vi "real time imaging v2.vi"() -> ()   [LabVIEW 2016]
uses:
  C:/Laser generated ultrasound/Labview/Kinesis Control/Thorlabs.MotionControl.KCube.BrushlessMotorCLI.dll
  Thorlabs.MotionControl.KCube.BrushlessMotorCLI.dll
  <vilib>/Analysis/3filter.llb/Filter Passband Type.ctl
  <vilib>/Analysis/baseanly.llb/Mean (DBL).vi
  <vilib>/Analysis/baseanly.llb/Real A x B.vi
  <vilib>/Utility/file.llb/Write To Spreadsheet File (DBL).vi
  <instrlib>/niScope/Acquire/Fetch/niScope Fetch.vi
  <vilib>/Analysis/Matrix/Numeric/Conversions/Array To Matrix - RA2.vi
  <vilib>/Analysis/Matrix/Numeric/Conversions/Matrix To Array - RM.vi
  <vilib>/Analysis/3filter.llb/Butterworth Filter (DBL).vi
  <instrlib>/niScope/Acquire/Fetch/niScope Multi Fetch.vi
  C:/Laser generated ultrasound/Labview/Kinesis Control/Thorlabs.MotionControl.Controls.dll
  Thorlabs.MotionControl.Controls.dll
  <vilib>/Analysis/NI_AALBase.lvlib
  <vilib>/Analysis/Matrix/NI_Matrix.lvlib
  <vilib>/Analysis/NI_AALPro.lvlib
panel:
  in  "stop":bool
  in  "Tab Control":T1(tab)
  in  "File Location":string="C:\\Laser generated ultrasound\\Labview\\Kinesis Control\\test data"
  in  "File name":string="scan_1"
  in  "SerialNumber":string="28251512"
  in  "Scan Length (mm)":dbl=20.0
  in  "Pullback speed (mm/s)":dbl=40.0
  in  "Repetition rate (Hz)":dbl=100.0
  in  "vertical range (V)":dbl=0.5 min=0.0 max=10.0 step=0.5
  in  "Depth (mm)":i32=15
  in  "Start acquisition":bool
  out "Number of samples":dbl
  out "number of a-lines":dbl
  in  "Apply frequency filter":bool
  in  "High Cutoff (MHz)":dbl=45.0
  in  "Low Cutoff (MHz)":dbl=1.0
  in  "Number of points":i32=150
  in  "Exponent":dbl=2.5
  out "spare a-lines":dbl
  out "?":cluster{dbl[], dbl[]}(graph)
  in  "Preview A-line?":bool
  in  "Start save":bool
  out "Intensity Graph":dbl[][](graph)
  in  "Stop save":bool
  out "Acquiring Data":bool
  in  "KCubeBrushlessControl":refnum<k24>(container)
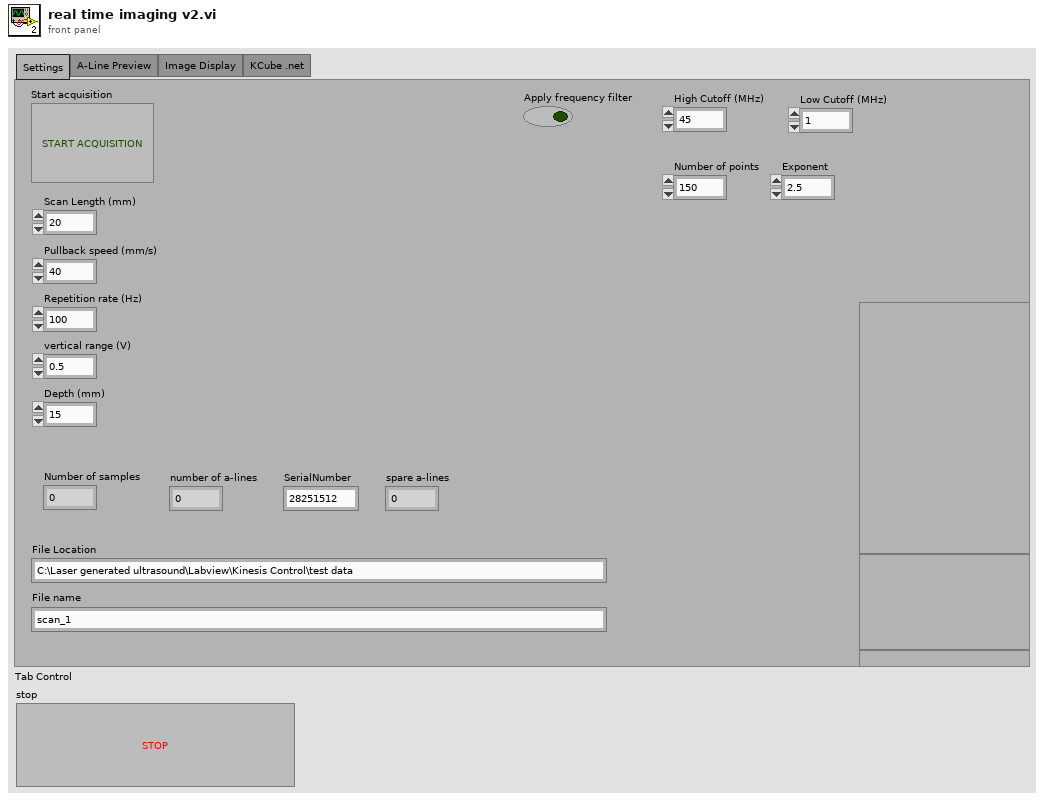
[diagram p1: front panel]
types:
  T1 = enum32{"Settings", "A-Line Preview", "Image Display", "KCube .net"}
  T2 = typedef "NI_AALBase.lvlib/Filter Passband Type.ctl" = enum32{"Lowpass", "Highpass", "Bandpass", "Bandstop"}
  T3 = typedef "NI_Matrix.lvlib/RealMatrix.ctl" = dbl[][]
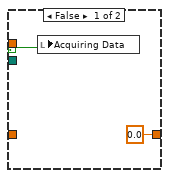
[diagram p8: hidden frame]
diagram:
  n1 = flat-sequence {
    tunnel: [w115] -> w72
    tunnel: [w114] -> w70
    tunnel: [w113] -> w68
    tunnel: [w111] -> w66
    tunnel: [w110] -> w64
    tunnel: [w98] -> w62
    tunnel: [w99] -> w60
    tunnel: ["Scan Length (mm)"] -> w58
    tunnel: ["Pullback speed (mm/s)"] -> w56
    tunnel: [w82] -> w54
    tunnel: ["File Location"] -> w53
    tunnel: ["File name"] -> w52
    tunnel: [w91] -> w44
    tunnel: [w91] -> w41
    tunnel: [w84] -> w11
    tunnel: ["Depth (mm)"] -> w6
    tunnel: [w82] -> w5
    tunnel: [w78] -> w4
    tunnel: [w77] -> w3
    tunnel: [w75] -> w2
    tunnel: [w73] -> w1
    tunnel: w72 -> [w181]
    tunnel: [w181] -> w71
    tunnel: w70 -> [w180]
    tunnel: [w180] -> w69
    tunnel: w68 -> [w179]
    tunnel: [w179] -> w67
    tunnel: w66 -> [w178]
    tunnel: [w178] -> w65
    tunnel: w64 -> [w177]
    tunnel: [w177] -> w63
    tunnel: w62 -> [w176]
    tunnel: [w176] -> w61
    tunnel: w60 -> [w175]
    tunnel: [w175] -> w59
    tunnel: w58 -> [w174]
    tunnel: [w174] -> w57
    tunnel: w56 -> [w173]
    tunnel: [w173] -> w55
    tunnel: w54 -> [w171]
    tunnel: w53 -> [w143]
    tunnel: w52 -> [w142]
    tunnel: w44 -> [w150]
    tunnel: [w150] -> w43
    tunnel: w41 -> [w148]
    tunnel: w11 -> [_]
    tunnel: [w136] -> w10
    tunnel: w6 -> [w140]
    tunnel: w5 -> [w139]
    tunnel: w4 -> [w135]
    tunnel: w3 -> [w134]
    tunnel: w2 -> [w133]
    tunnel: w1 -> [w130]
    tunnel: w71 -> [w194]
    tunnel: w69 -> [w189]
    tunnel: w67 -> [w190]
    tunnel: [w194] -> w51
    tunnel: [w189] -> w50
    tunnel: [w190] -> w49
    tunnel: w65 -> [w188]
    tunnel: w63 -> [w187]
    tunnel: [w188] -> w48
    tunnel: [w187] -> w47
    tunnel: [w186] -> w46
    tunnel: w61 -> [w185]
    tunnel: [w185] -> w45
    tunnel: w59 -> [w186]
    tunnel: w57 -> [_]
    tunnel: w55 -> [w184]
    tunnel: w43 -> [w183]
    tunnel: [w183] -> w42
    tunnel: w10 -> [w182]
    tunnel: [w182] -> w9
    tunnel: w51 -> [w207]
    tunnel: [w207] -> w40
    tunnel: w50 -> [w206]
    tunnel: [w206] -> w38
    tunnel: w49 -> [w205]
    tunnel: [w205] -> w36
    tunnel: w48 -> [w204]
    tunnel: [w203] -> w34
    tunnel: w47 -> [w202]
    tunnel: [w201] -> w32
    tunnel: w46 -> [w200]
    tunnel: [w197] -> w30
    tunnel: w45 -> [w199]
    tunnel: [w196] -> w28
    tunnel: w42 -> [w198]
    tunnel: w9 -> [w195]
    tunnel: [w195] -> w8
    tunnel: w40 -> [w237]
    tunnel: [w237] -> w39
    tunnel: w38 -> [w236]
    tunnel: [w236] -> w37
    tunnel: w36 -> [w235]
    tunnel: [w235] -> w35
    tunnel: w34 -> [w234]
    tunnel: [w234] -> w33
    tunnel: w32 -> [w233]
    tunnel: [w233] -> w31
    tunnel: w30 -> [w232]
    tunnel: [w230] -> w29
    tunnel: w28 -> [w231]
    tunnel: [w229] -> w27
    tunnel: [w225] -> w26
    tunnel: w8 -> [w224]
    tunnel: [w224] -> w7
    tunnel: w39 -> [w249]
    tunnel: w37 -> [w247]
    tunnel: w35 -> [w248]
    tunnel: [w249] -> w25
    tunnel: [w247] -> w23
    tunnel: [w248] -> w21
    tunnel: w33 -> [w246]
    tunnel: w31 -> [w245]
    tunnel: [w246] -> w19
    tunnel: [w245] -> w17
    tunnel: [w241] -> w15
    tunnel: [w240] -> w13
    tunnel: w29 -> [w244]
    tunnel: w27 -> [w243]
    tunnel: w26 -> [w242]
    tunnel: w7 -> [w239]
    tunnel: w25 -> [w543]
    tunnel: [w543] -> w24
    tunnel: w23 -> [w542]
    tunnel: [w542] -> w22
    tunnel: w21 -> [w541]
    tunnel: [w541] -> w20
    tunnel: w19 -> [w540]
    tunnel: [w540] -> w18
    tunnel: w17 -> [w539]
    tunnel: [w539] -> w16
    tunnel: w15 -> [w538]
    tunnel: [w538] -> w14
    tunnel: w13 -> [w537]
    tunnel: [w537] -> w12
    tunnel: w24 -> [w545]
    tunnel: w22 -> [w544]
    tunnel: w20 -> [_]
    tunnel: w18 -> [w549]
    tunnel: w16 -> [w548]
    tunnel: w14 -> [w547]
    tunnel: w12 -> [w546]
    frame #0 {
      # "spare a lines are acquired before the motor moves\nthink of this as a buffer to remove them\n0.05 estimated empirically"
      # "add extra a-lines as a buffer"
      # "calculate number of a-lines"
      # "Initiialise data array"
      # "round trip"
      # "speed of sound"
      # "convert depth to samples"
      # "convert to metre"
      # "Intialise all the equipment\n1. Motor\n2. Trigger\n3. Acquisition"
      n2 = Multiply(x=1500 ("y"), y=1e-08) -> (x*y=w103:dbl)
      n3 = local read "Pullback speed (mm/s)"() -> (w88:dbl)
      n4 = local read "Scan Length (mm)"() -> (w89:dbl)
      n5 = call "pulse_init.vi"("Repetition rate"="Repetition rate (Hz)") -> ("error out"=w110:errorcluster, "Refnum out"=w111:refnum<k21>)  [unwired: 9 in]
      n6 = local read "Repetition rate (Hz)"() -> (w87:dbl)
      n7 = Divide(x="Depth (mm)", y=1000) -> (x/y=w102:dbl)
      n8 = Multiply(x=w102, y=2.0) -> (x*y=w100:dbl)
      n9 = property class="KCubeBrushlessControl"(reference="KCubeBrushlessControl", "SerialNumber"="SerialNumber") -> (reference out=w119:refnum<k24>, error out=w118:errorcluster)  [unwired: 1 in]
      n10 = Divide(x=w100, y=w103) -> (x/y=w105:dbl)
      n11 = local read "Scan Length (mm)"() -> (w79:dbl)
      n12 = local read "Pullback speed (mm/s)"() -> (w77:dbl)
      n13 = Round Toward +Infinity(x=w105) -> (ceil(x): smallest int >= x=w82:dbl)
      "Number of samples" <- w82
      n14 = Initialize Array(0.0 ("element"), w82) -> (w92:dbl[])
      n15 = for {
        N: w82 -> [_]
        shift-right: [w127] -> w91
        shift-left: w92 -> [w126]
        i -> [w125]
        # "Create time axis"
        n16 = To Double Precision Float(number=w125) -> (double precision float=w124:dbl)
        n17 = Multiply(x=w124, y=1e-08) -> (x*y=w122:dbl)
        n18 = Replace Array Subset(array=w126, new element=w122, index=w125) -> (w127:dbl[])
      }
      n19 = Divide(x=w89, y=w88) -> (x/y=w86:dbl)
      n20 = local read "Repetition rate (Hz)"() -> (w75:dbl)
      n21 = Multiply(x=w86, y=w87) -> (x*y=w85:dbl)
      n22 = call "scope_init.vi"("Num Samples"=w82, "vertical range"="vertical range (V)", "Averages"=1) -> ("error out"=w98:errorcluster, "IVI Refnum out"=w99:refnum<k15>)  [unwired: 7 in]
      n23 = Initialize Array(0.0 ("element"), w82, w85) -> (w84:dbl[][])
      n24 = invoke class="KCubeBrushlessControl" method="CreateDevice"(reference=w119, error in=w118) -> (reference out=w117:refnum<k24>, error out=w116:errorcluster)  [unwired: 1 in, 1 out]
      n25 = Divide(x=w77, y=w75) -> (x/y=w80:dbl)
      n26 = Divide(x=w79, y=w80) -> (x/y=w81:dbl)
      n27 = Multiply(x=w75, y=0.05 ("x")) -> (x*y=w74:dbl)
      n28 = property class="KCubeBrushlessControl"(reference=w117, error in=w116) -> (reference out=w115:refnum<k24>, error out=w114:errorcluster, "Device"=w113:refnum<k24>)
      n29 = Round Toward +Infinity(x=w74) -> (ceil(x): smallest int >= x=w73:dbl)
      "spare a-lines" <- w73
      n30 = Add(x=w81, y=w73) -> (x+y=w78:dbl)
      "number of a-lines" <- w78
    }
    frame #1 {
      w128 = "\r"
      w131 = "\t"
      # "Calculate spare a-lines before move"
      # "Save the header file"
      # "Initialise the data matrix"
      # "Initialise the data matrix\nSave the Header file"
      n31 = local read "Repetition rate (Hz)"() -> (w158:dbl)
      n32 = local read "Number of samples"() -> (w164:dbl)
      n33 = local read "number of a-lines"() -> (w161:dbl)
      n34 = local read "Scan Length (mm)"() -> (w155:dbl)
      n35 = local read "Pullback speed (mm/s)"() -> (w152:dbl)
      n36 = Number To Decimal String(number=w164) -> (decimal integer string=w163:string)  [unwired: 1 in]
      n37 = Number To Decimal String(number=w158) -> (decimal integer string=w157:string)  [unwired: 1 in]
      n38 = Number To Decimal String(number=w161) -> (decimal integer string=w160:string)  [unwired: 1 in]
      n39 = Number To Decimal String(number=w155) -> (decimal integer string=w154:string)  [unwired: 1 in]
      n40 = Concatenate Strings(w143, "\\" ("string"), w142, "_hdr.txt" ("string")) -> (w169:string)
      n41 = Divide(x=w140, y=w139) -> (x/y=w138:dbl)
      n42 = Number To Decimal String(number=w152) -> (decimal integer string=w151:string)  [unwired: 1 in]
      n43 = Concatenate Strings(w143, "\\" ("string"), w142, "_taxis.txt" ("string")) -> (w147:string)
      n44 = Divide(x=w134, y=w133) -> (x/y=w141:dbl)
      n45 = String To Path(string=w147) -> (path=w144:path)
      n46 = property on="Intensity Graph" class="IntGraph (strict)"("XScale.Multiplier"=w141, "YScale.Multiplier"=w138) -> ()  [unwired: 2 in, 2 out]
      n47 = Number To Decimal String(number=w130) -> (decimal integer string=w129:string)  [unwired: 1 in]
      n48 = property on="Intensity Graph" class="IntGraph (strict)"("ZScale.MarkerVals[]"=cluster{dbl, u32}[] [{0.0, 0}, {-1.0, 16711680}, {-2.0, 16744192}, {-3.0, 16777087}, {-5.0, 16777215}] ("Z Scale.Marker Values[]")) -> ()  [unwired: 2 in, 2 out]
      n49 = Initialize Array(0.0 ("element"), w171, w135) -> (w136:dbl[][])
      n50 = call-poly <vilib>:"Write To Spreadsheet File.vi"("format (%.3f)"="%#g", "1D data"=w148, "file path (dialog if empty)"=w144) -> ()  [unwired: 5 in, 1 out]
      n51 = Concatenate Strings("Samples per A-line" ("string"), w131, w163, w128, "Number of A-lines" ("string"), w131, w160, w128, "Repetition rate (Hz)" ("string"), w131, w157, w128, "Scan length (mm)" ("string"), w131, w154, w128, "Pullback speed (mm/s)" ("string"), w131, w151, w128, "Spare a-line" ("string"), w131, w129, w128) -> (w166:string)
      n52 = String To Path(string=w169) -> (path=w170:path)
      n53 = Write to Text File(file (use dialog)=w170, text=w166) -> ()  [unwired: 2 in, 3 out]
    }
    frame #2 {
      # "Initial data array"
      # "Home the motor"
      n54 = invoke class="KCubeBrushlessMotor" method="Home"(reference=w190, error in=w189, "waitTimeout"=50000) -> ()  [unwired: 1 in, 4 out]
      n55 = invoke class="KCubeBrushlessMotor" method="SetVelocityParams"(reference=w190, error in=w189, "maxVelocity"=w184, "acceleration"=999.7) -> ()  [unwired: 1 in, 5 out]
      n56 = Wait (ms)(milliseconds to wait=u32 1000) -> ()  [unwired: 1 out]
    }
    frame #3 {
      # "A-line display for positioning"
      n57 = while {
        tunnel: w204 -> [w222]
        tunnel: w202 -> [w221]
        tunnel: [w222] -> w203
        tunnel: [w221] -> w201
        tunnel: w200 -> [w218]
        tunnel: w199 -> [w217]
        tunnel: w198 -> [w212]
        tunnel: [w209] -> w197
        tunnel: [w208] -> w196
        stop <- "Start acquisition" stop-if-true
        n58 = local read "Number of samples"() -> (w220:dbl)
        n59 = call <instrlib>:"niScope Initiate Acquisition.vi"("instrument handle"=w218, "error in"=w217) -> ("instrument handle out"=w216:refnum<k15>, "error out"=w215:errorcluster)  [unwired: 12 in]
        n60 = call-poly <instrlib>:"niScope Fetch (poly).vi"("error in"=w215, "numSamples"=w220, "channels"="0", "instrument handle"=w216) -> ("error out"=w208:errorcluster, "wfm"=w214:dbl[], "instrument handle out"=w209:refnum<k15>)  [unwired: 4 in, 1 out]
        n61 = Bundle(w212, "wfm"=w214) -> (w213:cluster{dbl[], "wfm":dbl[]})  [unwired: 1 in]
        n62 = case shown="True" "Preview A-line?" {
          tunnel: w213 -> [_ w223]
          frame False {
          }
          frame True {
            "?" <- w223
          }
        }
      }
    }
    frame #4 {
      # "Setup acquisition cards to record all a-lines"
      n63 = local read "Number of samples"() -> (w225:dbl)
      n64 = local read "number of a-lines"() -> (w226:dbl)
      n65 = call <instrlib>:"niScope Configure Horizontal Timing.vi"("instrument handle"=w232, "number of records"=w226, "min sample rate"=100000000.0, "reference position"=0.0, "error in"=w231, "min record length"=w225) -> ("instrument handle out"=w230:refnum<k15>, "error out"=w229:errorcluster)  [unwired: 8 in]
    }
    frame #5 {
      w238 = 0.0 ("y")
      # "move to end and acquire data\n1. move motor\n2. acquire data"
      n66 = while {
        tunnel: w248 -> [w291]
        tunnel: w247 -> [w290]
        tunnel: w242 -> [w287]
        shift-right: [w283] -> w241
        shift-left: w244 -> [w289]
        shift-right: [w282] -> w240
        shift-left: w243 -> [w288]
        shift-right: [w281] -> _
        shift-left: w239 -> [w280]
        shift-right: [w279] -> _
        shift-left: w238 -> [w278]
        shift-right: [w277] -> _
        shift-left: w238 -> [w276]
        shift-right: [w275] -> _
        shift-left: w238 -> [w274]
        stop <- "stop" stop-if-true
        # "Image number increment"
        # "Numeric to act as boolean to keep save going"
        n67 = call <instrlib>:"niScope Initiate Acquisition.vi"("instrument handle"=w289, "error in"=w288) -> ("instrument handle out"=w286:refnum<k15>, "error out"=w285:errorcluster)  [unwired: 12 in]
        n68 = flat-sequence {
          tunnel: w291 -> [w351]
          tunnel: w290 -> [w350]
          tunnel: w287 -> [w302]
          tunnel: w286 -> [w346]
          tunnel: w285 -> [w345]
          tunnel: [w349] -> w273
          tunnel: [w348] -> w271
          tunnel: [w299] -> w269
          tunnel: [w299] -> w267
          tunnel: [w341] -> w265
          tunnel: [w340] -> w263
          tunnel: w280 -> [w296]
          tunnel: [w298] -> w261
          tunnel: [w332] -> w259
          tunnel: w278 -> [w330]
          tunnel: w276 -> [w325]
          tunnel: [w324] -> w257
          tunnel: w274 -> [w323]
          tunnel: [w323] -> w255
          tunnel: ["Apply frequency filter"] -> w253
          tunnel: [w302] -> w251
          tunnel: w273 -> [w408]
          tunnel: [w406] -> w272
          tunnel: w271 -> [w407]
          tunnel: [w405] -> w270
          tunnel: w269 -> [w418]
          tunnel: [w418] -> w268
          tunnel: w267 -> [w417]
          tunnel: [w417] -> w266
          tunnel: w265 -> [w416]
          tunnel: [w416] -> w264
          tunnel: w263 -> [w415]
          tunnel: [w415] -> w262
          tunnel: w261 -> [w414]
          tunnel: [w414] -> w260
          tunnel: w259 -> [w413]
          tunnel: [w413] -> w258
          tunnel: w257 -> [w412]
          tunnel: [w412] -> w256
          tunnel: w255 -> [w411]
          tunnel: [w411] -> w254
          tunnel: w253 -> [w410]
          tunnel: [w410] -> w252
          tunnel: w251 -> [w409]
          tunnel: [w409] -> w250
          tunnel: [w464] -> w282
          tunnel: [w465] -> w283
          tunnel: w272 -> [w467]
          tunnel: w270 -> [w466]
          tunnel: w268 -> [w470]
          tunnel: w266 -> [w431]
          tunnel: w264 -> [w463]
          tunnel: w262 -> [w462]
          tunnel: w260 -> [w457]
          tunnel: [w424] -> w281
          tunnel: [w456] -> w279
          tunnel: w258 -> [w450]
          tunnel: w256 -> [w441]
          tunnel: [w454] -> w277
          tunnel: w254 -> [w449]
          tunnel: [w451] -> w275
          tunnel: w252 -> [w428]
          tunnel: w250 -> [w426]
          frame #0 {
            w309 = 20 ("length")
            # "Remove stationary a-lines"
            # "Frequency filter"
            # "cross-talk removal"
            # "Calculate the running average"
            # "take first few A-lines to repeat and use for running average"
            # "0 - 2000 - time\n1 - 50 - a-lines"
            # "NEXT STEPS:\n\nWork on the timing for motor movements"
            n69 = local read "Scan Length (mm)"() -> (w342:dbl)
            n70 = local read "spare a-lines"() -> (w294:dbl)
            n71 = local read "number of a-lines"() -> (w293:dbl)
            n72 = local read "Number of samples"() -> (w310:dbl)
            n73 = Number To Decimal String(number=w323) -> (decimal integer string=w322:string)  [unwired: 1 in]
            n74 = Number To Decimal String(number=w330) -> (decimal integer string=w320:string)  [unwired: 1 in]
            n75 = local read "File Location"() -> (w335:string)
            n76 = local read "File name"() -> (w333:string)
            n77 = Subtract(x=w293, y=w294) -> (x-y=w292:dbl)
            n78 = Delete From Array(array=w296, length=w294, index (col)=w292) -> (array with subset deleted=w295:dbl[][])  [unwired: 1 in, 1 out]
            n79 = invoke class="KCubeBrushlessMotor" method="MoveTo"(reference=w351, error in=w350, "position"=w342, "waitTimeout"=2000) -> (reference out=w341:refnum<k24>, error out=w340:errorcluster)  [unwired: 1 in, 3 out]
            n80 = Array Subset(array=w295, index (row)=0 ("index"), length (row)=w310, index (col)=0 ("index"), length (col)=w309) -> (w313:dbl[][])
            n81 = Concatenate Strings(w335, "\\" ("string"), w333, "_image_" ("string"), w322, "_f_" ("string"), w320, ".txt" ("string")) -> (w337:string)
            n82 = for {
              tunnel: w313 -> [w397] mode=indexing
              tunnel: [w396] -> w312 mode=indexing
              n83 = Reverse 1D Array(array=w397) -> (reversed array=w396:dbl[])
            }
            n84 = call-poly <instrlib>:"niScope Fetch (poly).vi"("timeout"=-1.0, "error in"=w345, "numSamples"=w302, "channels"="0", "instrument handle"=w346) -> ("error out"=w348:errorcluster, "wfm"=w317:dbl[][], "instrument handle out"=w349:refnum<k15>)  [unwired: 3 in, 1 out]
            n85 = String To Path(string=w337) -> (path=w336:path)
            n86 = Equal?(x=w325, y=1.0) -> (x = y?=w327:bool)
            n87 = Or(x="Start save", y=w327) -> (x .or. y?=w329:bool)
            n88 = local read "number of a-lines"() -> (w308:dbl)
            n89 = Insert Into Array(array=w295, index (col)=0 ("disabled index (col)"), new element=w312) -> (w311:dbl[][])  [unwired: 1 in]
            n90 = case shown="True" w329 {
              tunnel: w295 -> [_ w403]
              tunnel: w336 -> [_ w402]
              tunnel: [w400 w401] -> w332
              tunnel: w330 -> [w400 w401]
              frame False {
              }
              frame True {
                n91 = call-poly <vilib>:"Write To Spreadsheet File.vi"("format (%.3f)"="%#g", "2D data"=w403, "file path (dialog if empty)"=w402) -> ()  [unwired: 5 in, 1 out]
              }
            }
            n92 = for {
              N: w308 -> [_]
              tunnel: w311 -> [w393]
              tunnel: w310 -> [w391]
              tunnel: w309 -> [w389]
              tunnel: [w387] -> w307 mode=indexing
              i -> [w390]
              n93 = Array Subset(array=w393, index (row)=0 ("index"), length (row)=w391, index (col)=w390, length (col)=w389) -> (w388:dbl[][])
              n94 = for {
                tunnel: w388 -> [w395] mode=indexing
                tunnel: [w394] -> w387 mode=indexing
                n95 = call-poly <vilib>:"Mean.vi"("X"=w395) -> ("mean"=w394:dbl)  [unwired: 1 out]
              }
            }
            n96 = Transpose 2D Array(2D array=w317) -> (transposed array=w300:dbl[][])
            n97 = case shown="True" "Start save" {
              tunnel: w325 -> [w398 _]
              tunnel: [w398 1.0 ("y")] -> w324
              frame False {
              }
              frame True {
              }
            }
            n98 = Transpose 2D Array(2D array=w295) -> (transposed array=w306:dbl[][])
            n99 = Replace Array Subset(array=w296, new element=w300, index (row)=0, index (col)=0 ("disabled index (col)")) -> (w298:dbl[][])
            n100 = for {
              N: w308 -> [_]
              tunnel: w307 -> [w380] mode=indexing
              tunnel: w306 -> [w379] mode=indexing
              tunnel: [w377] -> w305 mode=indexing
              n101 = call "create_design_matrix.vi"("input vector"=w380) -> ("design matrix"=w386:dbl[][])
              n102 = Array Size(array=w379) -> (size(s)=w381:i32)
              n103 = call "linear_fit.vi"("Real 1D Array"=w379, "X"=w386) -> ("A x B"=w385:T3)
              n104 = call-poly <vilib>:"Array To Matrix.vi"("Real 2D Array"=w386) -> ("Real Matrix"=w384:T3)
              n105 = call-poly <vilib>:"A x B.vi"("B"=w384, "A"=w385) -> ("A x B"=w383:T3)  [unwired: 1 out]
              n106 = call-poly <vilib>:"Matrix To Array.vi"("Real Matrix"=w383) -> ("Real 2D Array"=w382:dbl[][])
              n107 = Reshape Array(w382, w381) -> (w378:dbl[])
              n108 = Subtract(x=w379, y=w378) -> (x-y=w377:dbl[])
            }
            n109 = Wait (ms)(milliseconds to wait=u32 5) -> ()  [unwired: 1 out]
            n110 = Delete From Array(array=w298, length=w294, index (col)=0 ("disabled index (col)")) -> (array with subset deleted=w299:dbl[][])  [unwired: 1 in, 1 out]
            n111 = case shown="True" "Apply frequency filter" {
              tunnel: w305 -> [w359 w361]
              tunnel: [w359 w360] -> w304
              frame False {
              }
              frame True {
                n112 = Multiply(x="High Cutoff (MHz)", y=1000000.0) -> (x*y=w367:dbl)
                n113 = Multiply(x="Low Cutoff (MHz)", y=1000000.0) -> (x*y=w366:dbl)
                n114 = for {
                  tunnel: 100000000.0 ("y") -> [w373]
                  tunnel: w367 -> [w372]
                  tunnel: w366 -> [w371]
                  tunnel: w361 -> [w370] mode=indexing
                  tunnel: [w369] -> w360 mode=indexing
                  n115 = call-poly <vilib>:"Butterworth Filter.vi"("init/cont (init:F)"=FALSE, "order"=8, "filter type"=Filter_Passband_Type."Bandpass", "low cutoff freq: fl"=w371, "high cutoff freq: fh"=w372, "sampling freq: fs"=w373, "X"=w370) -> ("Filtered X"=w369:dbl[])  [unwired: 1 in, 1 out]
                }
              }
            }
            n116 = for {
              tunnel: w304 -> [w358] mode=indexing
              tunnel: [w352] -> w301 mode=indexing
              n117 = call <vilib>:"Fast Hilbert Transform.vi"("X"=w358) -> ("Hilbert{X}"=w357:dbl[])  [unwired: 1 out]
              n118 = Absolute Value(x=w357) -> (abs(x)=w356:dbl[])
              n119 = call "TGC_exponential.vi"("Exponent"="Exponent", "Number of points"="Number of points", "Input vector"=w356) -> ("Output vector"=w353:dbl[])
              n120 = Logarithm Base 10(1:w353) -> (0:w352:dbl[])
            }
            n121 = local write "Intensity Graph"(w301) -> ()
          }
          frame #1 {
            n122 = call <instrlib>:"niScope Initiate Acquisition.vi"("instrument handle"=w408, "error in"=w407) -> ("instrument handle out"=w406:refnum<k15>, "error out"=w405:errorcluster)  [unwired: 12 in]
          }
          frame #2 {
            w436 = 20 ("length")
            # "reverse array direction to match"
            # "Frequency filter"
            # "cross-talk removal"
            # "Calculate the running average"
            n123 = local read "File name"() -> (w471:string)
            n124 = local read "File Location"() -> (w472:string)
            n125 = Number To Decimal String(number=w449) -> (decimal integer string=w447:string)  [unwired: 1 in]
            n126 = Number To Decimal String(number=w450) -> (decimal integer string=w445:string)  [unwired: 1 in]
            n127 = invoke class="KCubeBrushlessMotor" method="MoveTo"(reference=w463, error in=w462, "position"=0.0, "waitTimeout"=2000) -> ()  [unwired: 1 in, 5 out]
            n128 = Concatenate Strings(w472, "\\" ("string"), w471, "_image_" ("string"), w447, "_b_" ("string"), w445, ".txt" ("string")) -> (w475:string)
            n129 = local read "Number of samples"() -> (w435:dbl)
            n130 = String To Path(string=w475) -> (path=w473:path)
            n131 = call-poly <instrlib>:"niScope Fetch (poly).vi"("timeout"=-1.0, "error in"=w466, "numSamples"=w426, "channels"="0", "instrument handle"=w467) -> ("error out"=w464:errorcluster, "wfm"=w442:dbl[][], "instrument handle out"=w465:refnum<k15>)  [unwired: 3 in, 1 out]
            n132 = Equal?(x=1.0, y=w441) -> (x = y?=w453:bool)
            n133 = local read "number of a-lines"() -> (w421:dbl)
            n134 = local read "spare a-lines"() -> (w420:dbl)
            n135 = case shown="True" w453 {
              selector: w453 -> [w529 w531]
              tunnel: w470 -> [_ w535]
              tunnel: w473 -> [_ w534]
              tunnel: w450 -> [_ w533]
              tunnel: [0.0 w532] -> w456
              frame False {
                n136 = local write "Acquiring Data"(w529) -> ()
              }
              frame True {
                n137 = call-poly <vilib>:"Write To Spreadsheet File.vi"("format (%.3f)"="%#g", "2D data"=w535, "file path (dialog if empty)"=w534) -> ()  [unwired: 5 in, 1 out]
                n138 = Increment(x=w533) -> (x+1=w532:dbl)
                "Acquiring Data" <- w531
              }
            }
            n139 = Array Subset(array=w431, index (row)=0 ("index"), length (row)=w435, index (col)=0 ("index"), length (col)=w436) -> (w434:dbl[][])
            n140 = Transpose 2D Array(2D array=w442) -> (transposed array=w423:dbl[][])
            n141 = for {
              tunnel: w434 -> [w514] mode=indexing
              tunnel: [w513] -> w433 mode=indexing
              n142 = Reverse 1D Array(array=w514) -> (reversed array=w513:dbl[])
            }
            n143 = Subtract(x=w421, y=w420) -> (x-y=w419:dbl)
            n144 = Wait (ms)(milliseconds to wait=u32 5) -> ()  [unwired: 1 out]
            n145 = Insert Into Array(array=w431, index (col)=0 ("disabled index (col)"), new element=w433) -> (w437:dbl[][])  [unwired: 1 in]
            n146 = for {
              N: w419 -> [_]
              tunnel: w437 -> [w521]
              tunnel: w435 -> [w519]
              tunnel: w436 -> [w517]
              tunnel: [w515] -> w432 mode=indexing
              i -> [w518]
              n147 = Array Subset(array=w521, index (row)=0 ("index"), length (row)=w519, index (col)=w518, length (col)=w517) -> (w516:dbl[][])
              n148 = for {
                tunnel: w516 -> [w523] mode=indexing
                tunnel: [w522] -> w515 mode=indexing
                n149 = call-poly <vilib>:"Mean.vi"("X"=w523) -> ("mean"=w522:dbl)  [unwired: 1 out]
              }
            }
            n150 = for {
              tunnel: w423 -> [w477] mode=indexing
              tunnel: [w476] -> w422 mode=indexing
              n151 = Reverse 1D Array(array=w477) -> (reversed array=w476:dbl[])
            }
            n152 = case shown="True" "Stop save" {
              tunnel: w441 -> [w525 _]
              tunnel: [w525 0.0 ("y")] -> w454
              tunnel: w449 -> [w524 w527]
              tunnel: [w524 w526] -> w451
              frame False {
              }
              frame True {
                n153 = Increment(x=w527) -> (x+1=w526:dbl)
              }
            }
            n154 = Transpose 2D Array(2D array=w431) -> (transposed array=w430:dbl[][])
            n155 = for {
              N: w419 -> [_]
              tunnel: w432 -> [w506] mode=indexing
              tunnel: w430 -> [w505] mode=indexing
              tunnel: [w503] -> w429 mode=indexing
              n156 = call "create_design_matrix.vi"("input vector"=w506) -> ("design matrix"=w512:dbl[][])
              n157 = Array Size(array=w505) -> (size(s)=w507:i32)
              n158 = call "linear_fit.vi"("Real 1D Array"=w505, "X"=w512) -> ("A x B"=w511:T3)
              n159 = call-poly <vilib>:"Array To Matrix.vi"("Real 2D Array"=w512) -> ("Real Matrix"=w510:T3)
              n160 = call-poly <vilib>:"A x B.vi"("B"=w510, "A"=w511) -> ("A x B"=w509:T3)  [unwired: 1 out]
              n161 = call-poly <vilib>:"Matrix To Array.vi"("Real Matrix"=w509) -> ("Real 2D Array"=w508:dbl[][])
              n162 = Reshape Array(w508, w507) -> (w504:dbl[])
              n163 = Subtract(x=w505, y=w504) -> (x-y=w503:dbl[])
            }
            n164 = Replace Array Subset(array=w457, new element=w422, index (row)=0, index (col)=0 ("disabled index (col)")) -> (w424:dbl[][])
            n165 = case shown="True" w428 {
              tunnel: w429 -> [w485 w489]
              tunnel: [w485 w488] -> w427
              frame False {
              }
              frame True {
                n166 = local read "High Cutoff (MHz)"() -> (w487:dbl)
                n167 = local read "Low Cutoff (MHz)"() -> (w486:dbl)
                n168 = Multiply(x=w487, y=1000000.0) -> (x*y=w493:dbl)
                n169 = Multiply(x=w486, y=1000000.0) -> (x*y=w492:dbl)
                n170 = for {
                  tunnel: 100000000.0 ("y") -> [w499]
                  tunnel: w493 -> [w498]
                  tunnel: w492 -> [w497]
                  tunnel: w489 -> [w496] mode=indexing
                  tunnel: [w495] -> w488 mode=indexing
                  n171 = call-poly <vilib>:"Butterworth Filter.vi"("init/cont (init:F)"=FALSE, "order"=8, "filter type"=Filter_Passband_Type."Bandpass", "low cutoff freq: fl"=w497, "high cutoff freq: fh"=w498, "sampling freq: fs"=w499, "X"=w496) -> ("Filtered X"=w495:dbl[])  [unwired: 1 in, 1 out]
                }
              }
            }
            n172 = for {
              tunnel: w427 -> [w484] mode=indexing
              tunnel: [w480] -> w425 mode=indexing
              n173 = local read "Number of points"() -> (w479:i32)
              n174 = call <vilib>:"Fast Hilbert Transform.vi"("X"=w484) -> ("Hilbert{X}"=w483:dbl[])  [unwired: 1 out]
              n175 = local read "Exponent"() -> (w478:dbl)
              n176 = Absolute Value(x=w483) -> (abs(x)=w482:dbl[])
              n177 = call "TGC_exponential.vi"("Exponent"=w478, "Number of points"=w479, "Input vector"=w482) -> ("Output vector"=w481:dbl[])
              n178 = Logarithm Base 10(1:w481) -> (0:w480:dbl[])
            }
            n179 = local write "Intensity Graph"(w425) -> ()
          }
        }
      }
    }
    frame #6 {
      # "Save data"
    }
    frame #7 {
      # "Close everything"
      n180 = call <vilib>:"DAQmx Stop Task.vi"("task/channels in"=w549, "error in"=w548) -> ("task out"=w551:refnum<k21>, "error out"=w550:errorcluster)  [unwired: 12 in]
      n181 = call <instrlib>:"niScope Close.vi"("instrument handle"=w547, "error in"=w546) -> ()  [unwired: 13 in, 1 out]
      n182 = call <vilib>:"DAQmx Clear Task.vi"("task in"=w551, "error in"=w550) -> ()  [unwired: 13 in, 1 out]
      n183 = invoke class="KCubeBrushlessControl" method="CloseDevice"(reference=w545, error in=w544) -> ()  [unwired: 1 in, 3 out]
    }
  }
